vi "HP 436A Read Single Measurement.vi"(10 "Mode":u8(ring)=68 items=["Watt"=65, "dB (Rel)"=66, "dB [Ref]"=67, "dBm"=68]) -> (3 "Measurement":dbl format="%#_6p")   [LabVIEW 2014]
doc: "Description:\nThis example shows how to use the HP 436A power meter driver to configure the meter and take a measurement.\n\nNotes:\n\n(1) This only works with HP 436A meters with option 022, HPIB."
uses:
  <instrlib>/HP 436A/HP 436A.lvlib
panel:
  in  "10 Sec Settling Time on Range 1?":bool=TRUE
  out "Range (1 is Most Sensitive)":u8
  in  "Reset Meter?":bool
  in  "Return to local mode?":bool
  out "Under Range":bool
  out "Reading Valid":bool
  out "Over Range":bool
  out "Units":string
  in  "Measurement Rate":u8(ring)=86 items=["Hold"=72, "Trigger with settling time"=84, "Trigger, immediate"=73, "Free Run at maximum rate"=82, "Free Run with settling time"=86]
  in  "Range":u8(ring)=9 items=["5 (Least Sensitive)"=5, "4"=4, "3"=3, "2"=2, "1 (Most Sensitive)"=1, "Auto"=9]
  in  "Enable Cal Factor":bool=TRUE
  in  "VISA resource name":refnum<visa-resource-name>="GPIB0::13::INSTR"
  # "(c) 2016 Matthew D'Asaro under the terms of the GPL v2"
  # "(Turn this on if the meter is not already in remote mode)"
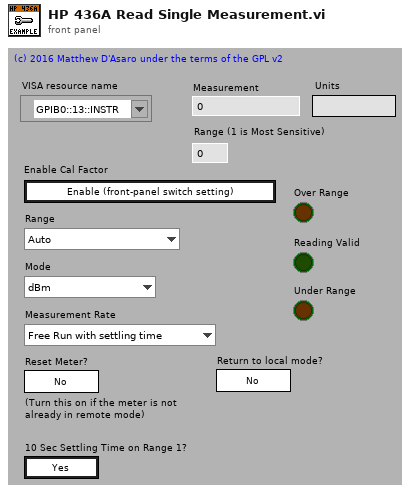
[diagram p1: front panel]
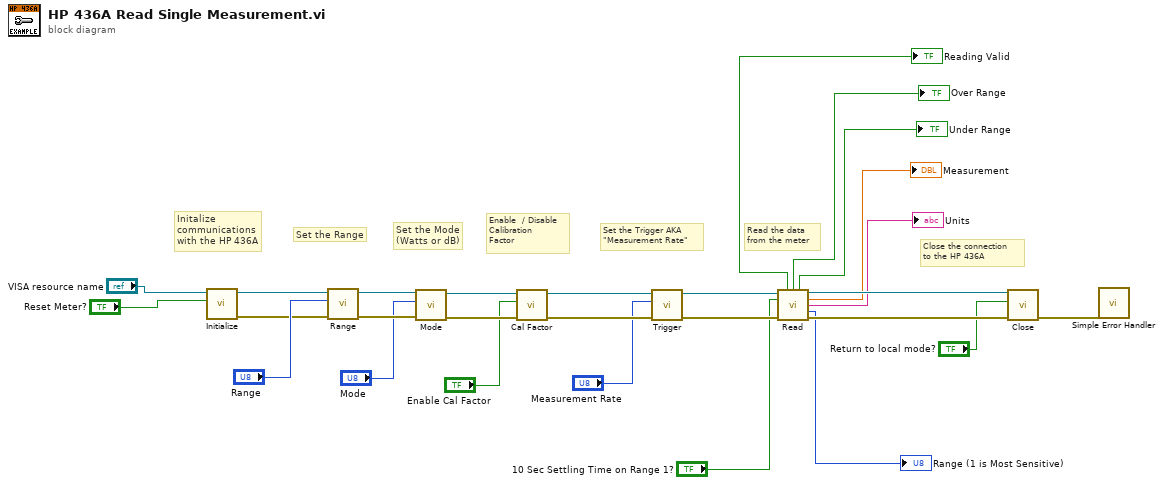
[diagram p0: block diagram]
diagram:
  # "Read the data\nfrom the meter"
  # "Close the connection\nto the HP 436A"
  # "Initalize\ncommunications\nwith the HP 436A"
  # "Set the Trigger AKA\n\"Measurement Rate\""
  # "Enable  / Disable\nCalibration\nFactor"
  # "Set the Mode\n(Watts or dB)"
  # "Set the Range"
  n1 = call <instrlib>:"Initialize.vi"("Reset Instrument?"="Reset Meter?", "VISA resource name"="VISA resource name") -> ("error out"=w7:errorcluster, "VISA resource name out"=w6:refnum<visa-resource-name>)  [unwired: 8 in]
  n2 = call <instrlib>:"Range.vi"("error in (no error)"=w7, "Range"="Range", "VISA resource name"=w6) -> ("error out"=w26:errorcluster, "VISA resource name out"=w27:refnum<visa-resource-name>)  [unwired: 7 in]
  n3 = call <instrlib>:"Mode.vi"("error in (no error)"=w26, "Mode"="Mode", "VISA resource name"=w27) -> ("error out"=w24:errorcluster, "VISA resource name out"=w25:refnum<visa-resource-name>)  [unwired: 7 in]
  n4 = call <instrlib>:"Cal Factor.vi"("error in (no error)"=w24, "Enable Cal Factor"="Enable Cal Factor", "VISA resource name"=w25) -> ("error out"=w22:errorcluster, "VISA resource name out"=w23:refnum<visa-resource-name>)  [unwired: 7 in]
  n5 = call <instrlib>:"Trigger.vi"("error in (no error)"=w22, "Measurement Rate"="Measurement Rate", "VISA resource name"=w23) -> ("error out"=w5:errorcluster, "VISA resource name out"=w17:refnum<visa-resource-name>)  [unwired: 7 in]
  n6 = call <instrlib>:"Read.vi"("VISA resource name"=w17, "10 Sec Settling Time on Range 1?"="10 Sec Settling Time on Range 1?", "error in (no error)"=w5) -> ("Reading Valid"=→"Reading Valid":bool, "Over Range"=→"Over Range":bool, "Under Range"=→"Under Range":bool, "VISA resource name out"=w16:refnum<visa-resource-name>, "Measurement"=→"Measurement":dbl, "Units"=→"Units":string, "Range (1-5 Where 1 is Most Sensitive)"=→"Range (1 is Most Sensitive)":u8, "error out"=w15:errorcluster)  [unwired: 2 in, 3 out]
  n7 = call <instrlib>:"Close.vi"("error in (no error)"=w15, "Return to local mode?"="Return to local mode?", "VISA resource name"=w16) -> ("error out"=w1:errorcluster)  [unwired: 8 in]
  n8 = call <vilib>:"Simple Error Handler.vi"("error in (no error)"=w1) -> ()  [unwired: 4 in, 5 out]
